vi "Read EEPROM User Area.vi"(8 "error in (no error)":errorcluster, 11 "Handle":u64) -> (0 "error out":errorcluster, 1 "Bytes Read":u32, 2 "User Area Data":u8[](array[numeric]) format="%x", 3 "Handle out":u64)   [LabVIEW 2019, in "D2XX-lv.lvlib"]
doc: "Read data from the EEPROM user area."
uses:
  D2XX-lv.lvlib
  <instrlib>/_D2XX/D2XX/D2XX.lvlib
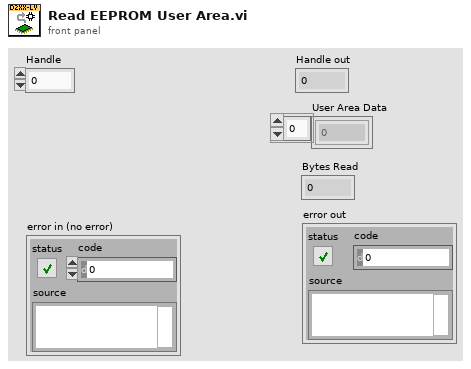
[diagram p1: front panel]
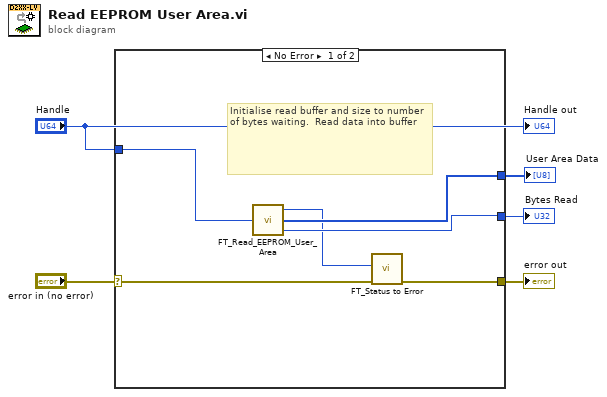
[diagram p0: block diagram]
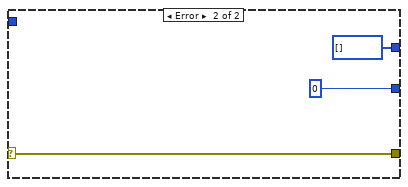
[diagram p2: hidden frame]
diagram:
  n1 = case shown="No Error" "error in (no error)" {
    selector: "error in (no error)" -> [w11 w14]
    tunnel: [w10 w14] -> w4
    tunnel: "Handle" -> [w9 _]
    tunnel: [w7 u32 0 ("Bytes Written")] -> w3
    tunnel: [w8 u8[] [] ("Read Data")] -> w1
    frame No Error {
      # "Initialise read buffer and size to number of bytes waiting.  Read data into buffer"
      n2 = call <instrlib>:"FT_Read_EEPROM_User_Area.vi"("Handle"=w9) -> ("FT_Status"=w6:u32, "User Area Data"=w8:u8[], "Bytes Read"=w7:u32)
      n3 = call "FT_Status to Error.vi"("error in (no error)"=w11, "FT_Status"=w6) -> ("error out"=w10:errorcluster)  [unwired: 9 in]
    }
    frame Error {
    }
  }
  "error out" <- w4
  "Bytes Read" <- w3
  "User Area Data" <- w1
  "Handle out" <- "Handle"
